vi "Fc_MenuSelections.vi"(6 "Cluster References":T2, 7 "ItemTag":string, 8 "error in (no error)":errorcluster, 9 "Cluster in":T1, 10 "VI caller":refnum<vi>, 11 "WaveformGraph in":refnum<vi>) -> (0 "error out":errorcluster, 3 "Cluster out":T1)   [LabVIEW 2021]
doc: "This function is used to select possible selection in the current window plot."
uses:
  <vilib>/Analysis/NI_AALBase.lvlib
  <vilib>/gmath/NI_Gmath.lvlib
  <vilib>/Analysis/1siggen.llb/Ramp Pattern by Samples.vi
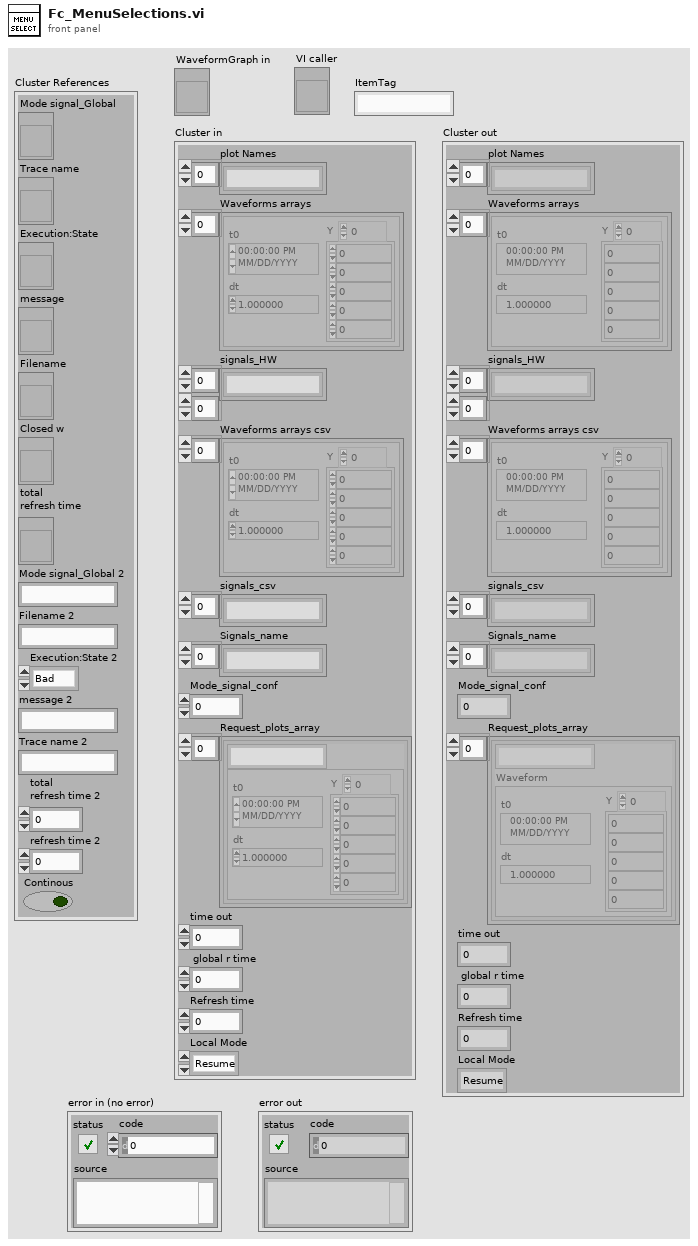
[diagram p1: front panel]
types:
  T1 = cluster{"plot Names":string[], "Waveforms arrays":waveform(dbl)[], "signals_HW":string[][], "Waveforms arrays csv":waveform(dbl)[], "signals_csv":string[], "Signals_name":string[], "Mode_signal_conf":u8, "Request_plots_array":cluster{string, "Waveform":waveform(dbl)}[], "time out":i32, " global r time":u32, "Refresh time":u32, "Local Mode":enum32{"Resume", "Hold"}}
  T2 = cluster{"Mode signal_Global":refnum<vi>, "Trace name":refnum<vi>, "Execution:State":refnum<vi>, "message":refnum<vi>, "Filename":refnum<vi>, "Closed w":refnum<vi>, "total \nrefresh time":refnum<vi>, "Mode signal_Global 2":string, "Filename 2":string, "Execution:State 2":enum32{"Bad", "Idle", "Run top level", "Running"}, "message 2":string, "Trace name 2":string, "total \nrefresh time 2":i32, "refresh time 2":i32, "Continous":bool}
  T3 = enum32{"Bad", "Idle", "Run top level", "Running"}
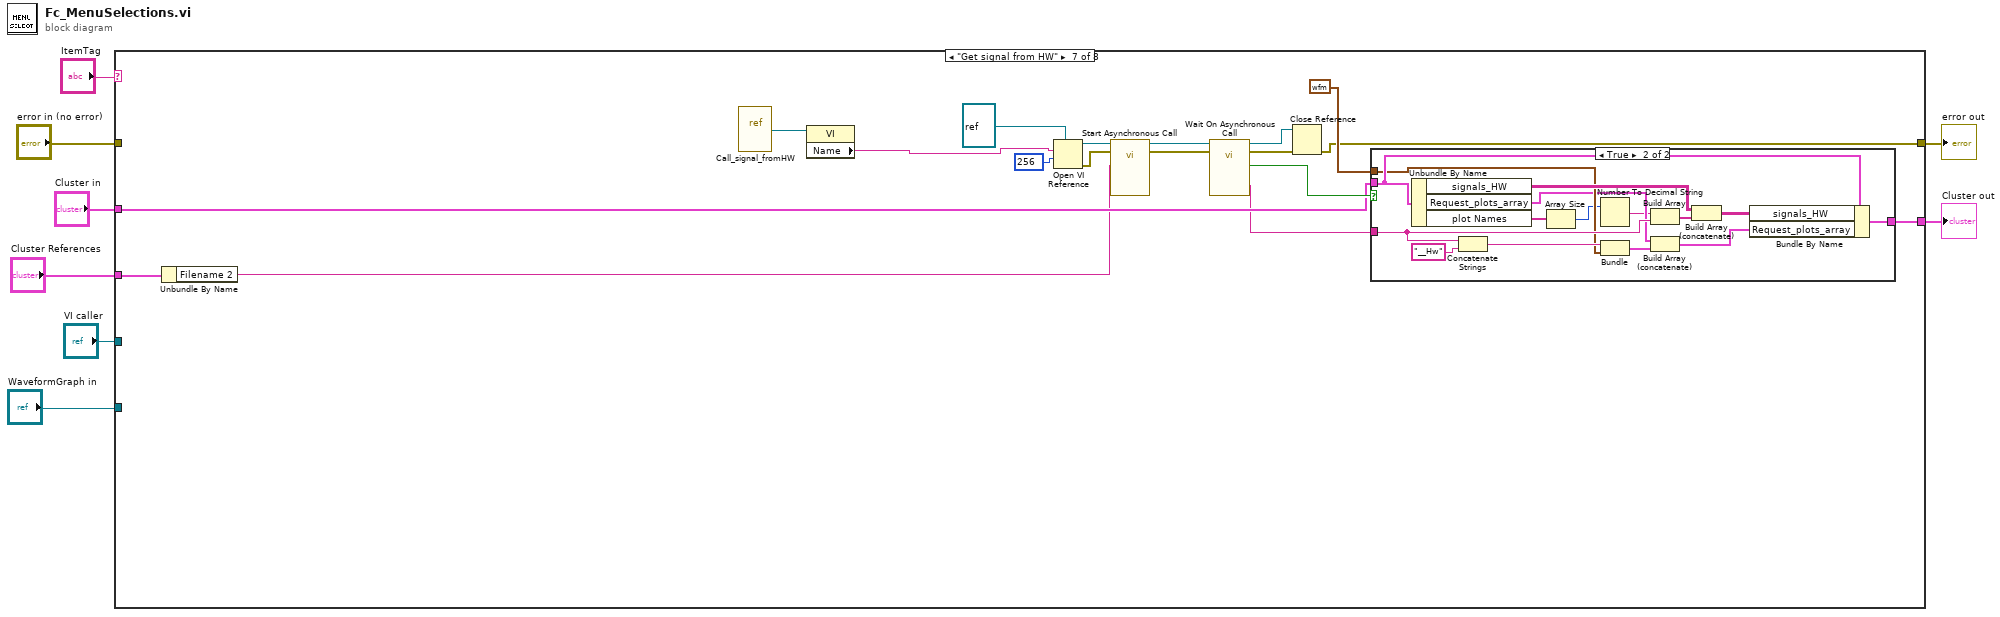
[diagram p0: block diagram]
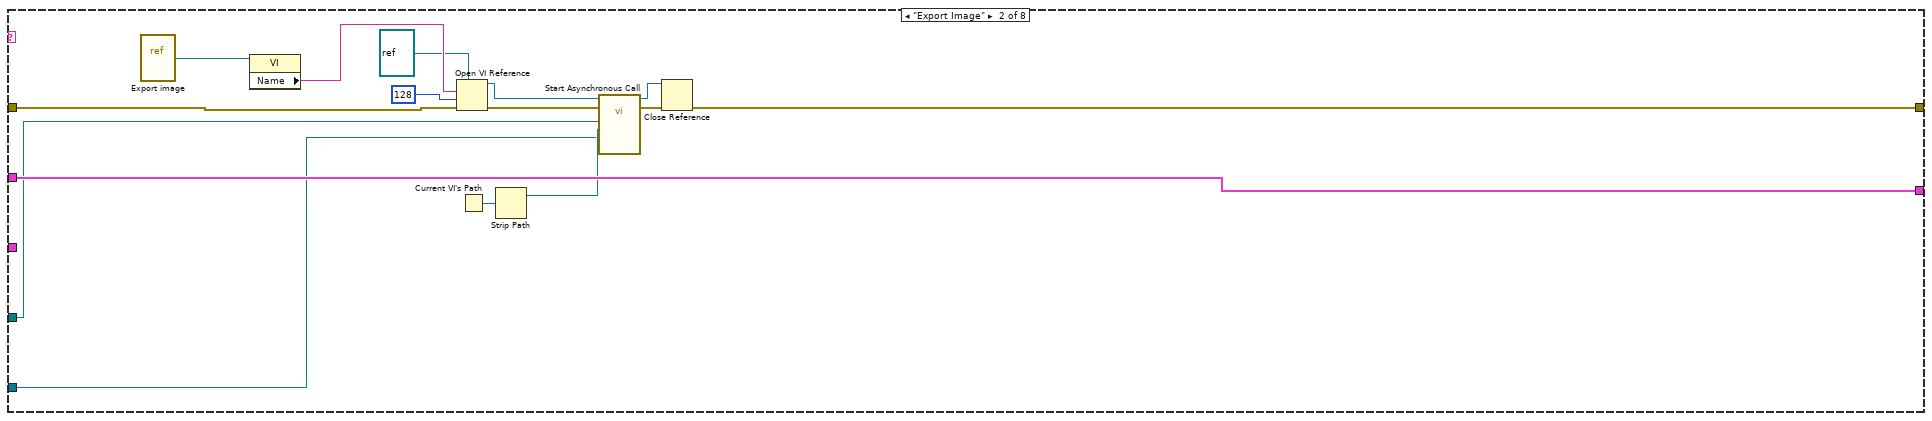
[diagram p3: hidden frame]
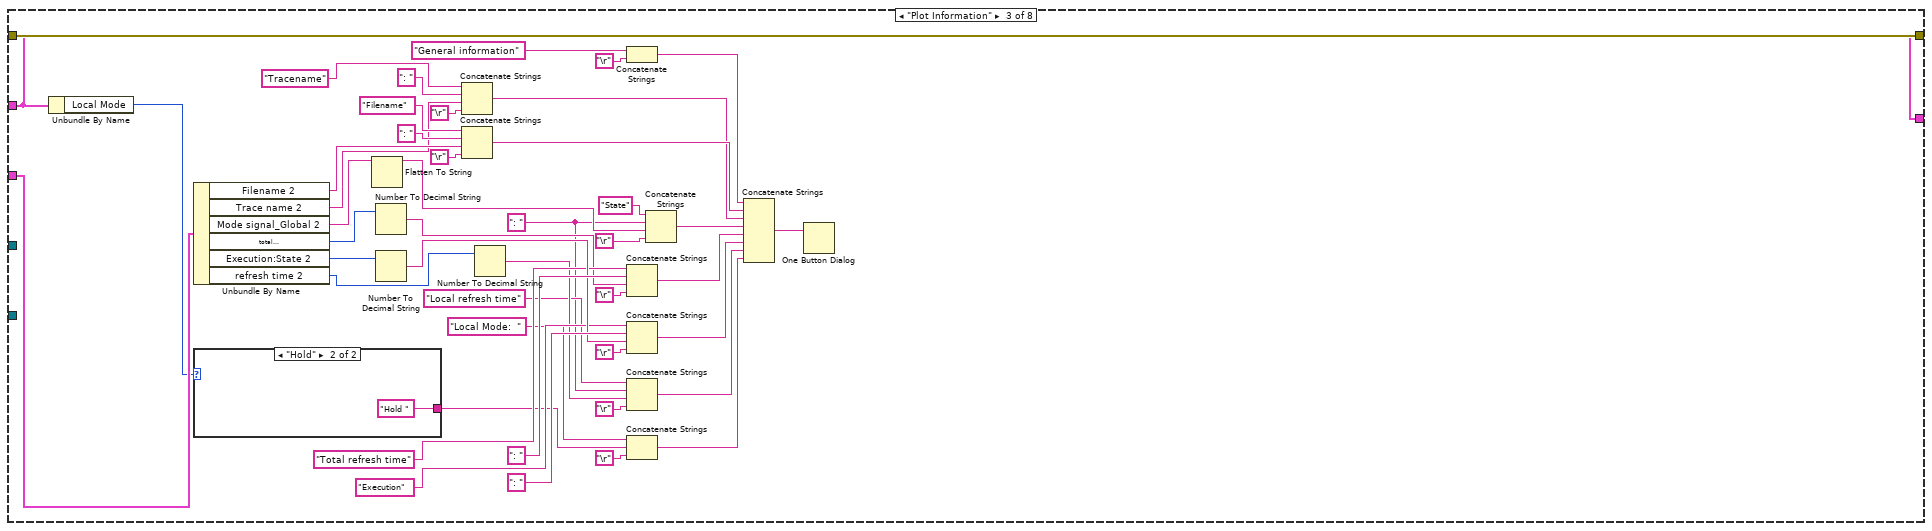
[diagram p4: hidden frame]
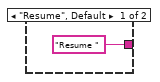
[diagram p5: hidden frame]
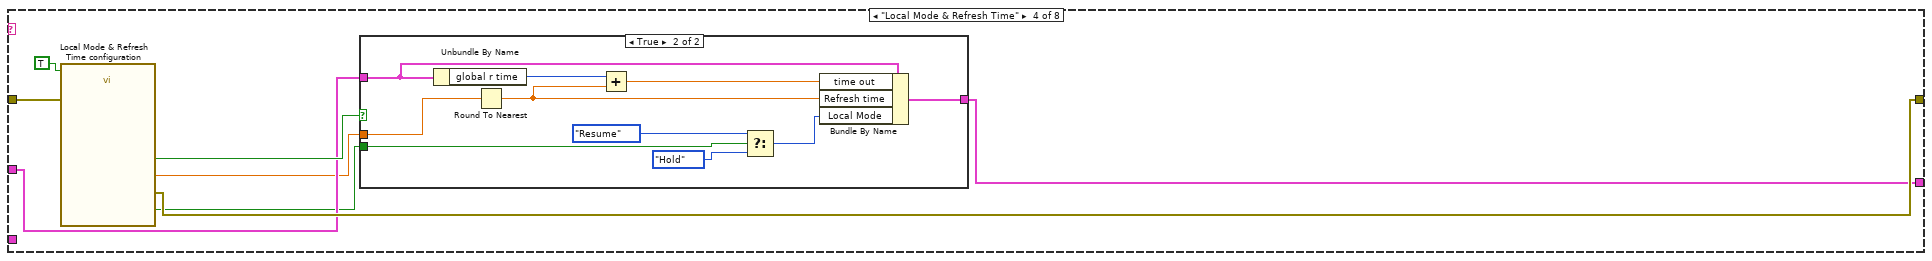
[diagram p6: hidden frame]
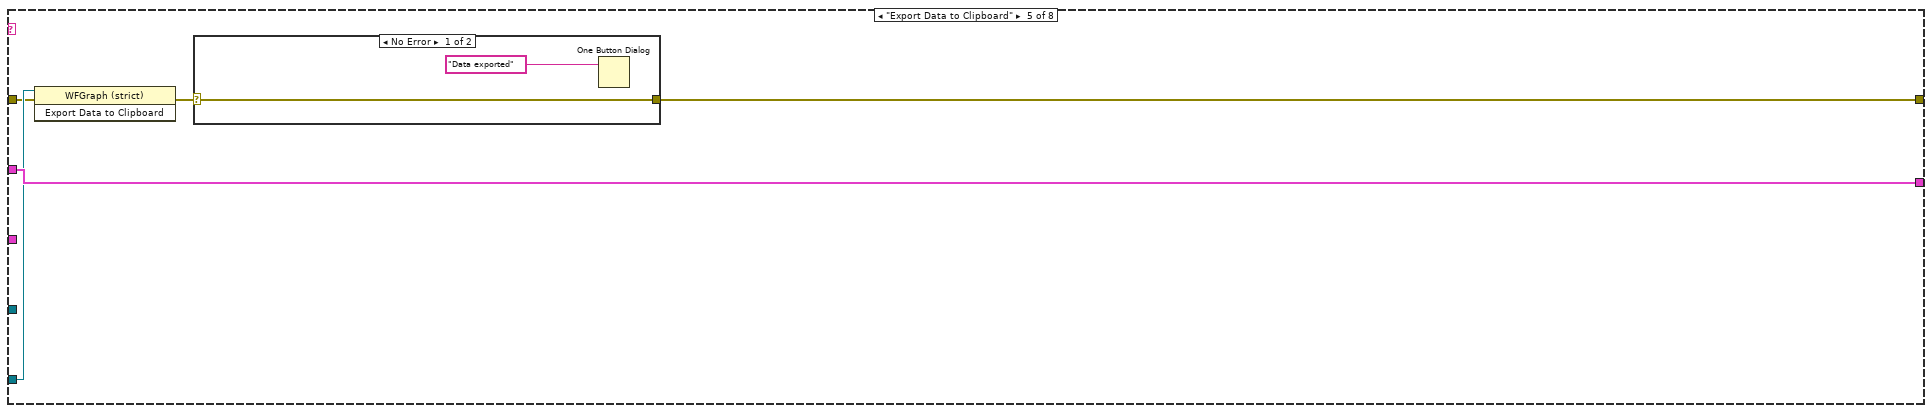
[diagram p8: hidden frame]
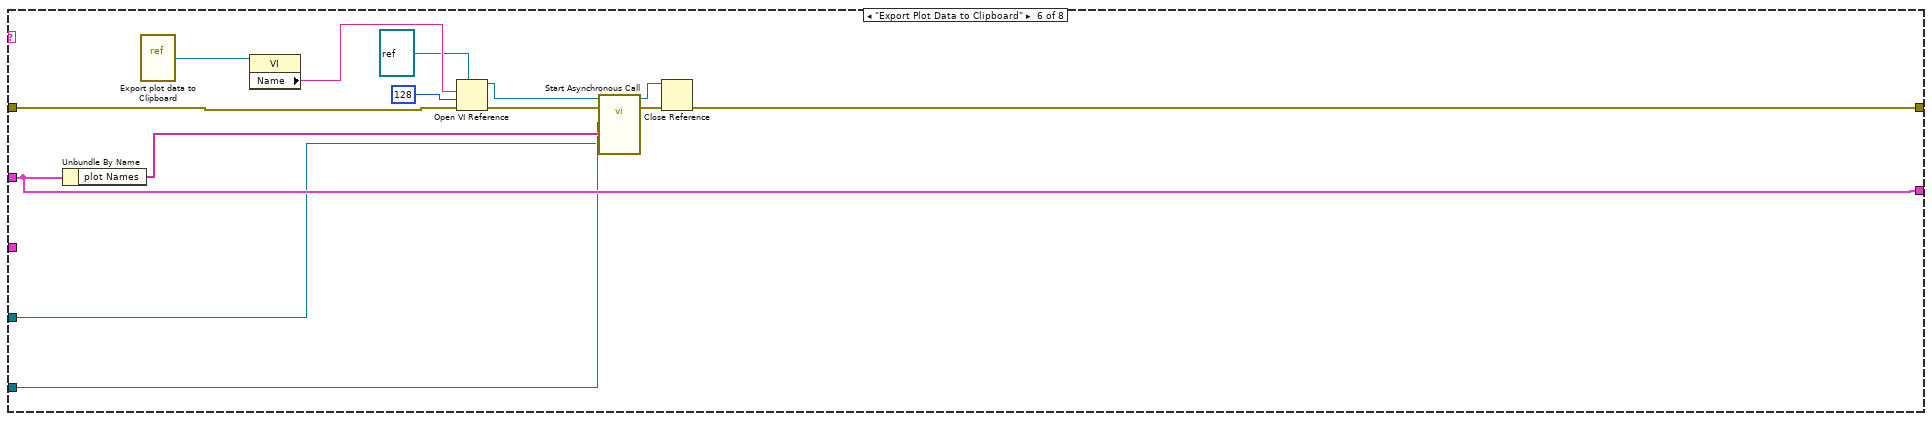
[diagram p10: hidden frame]
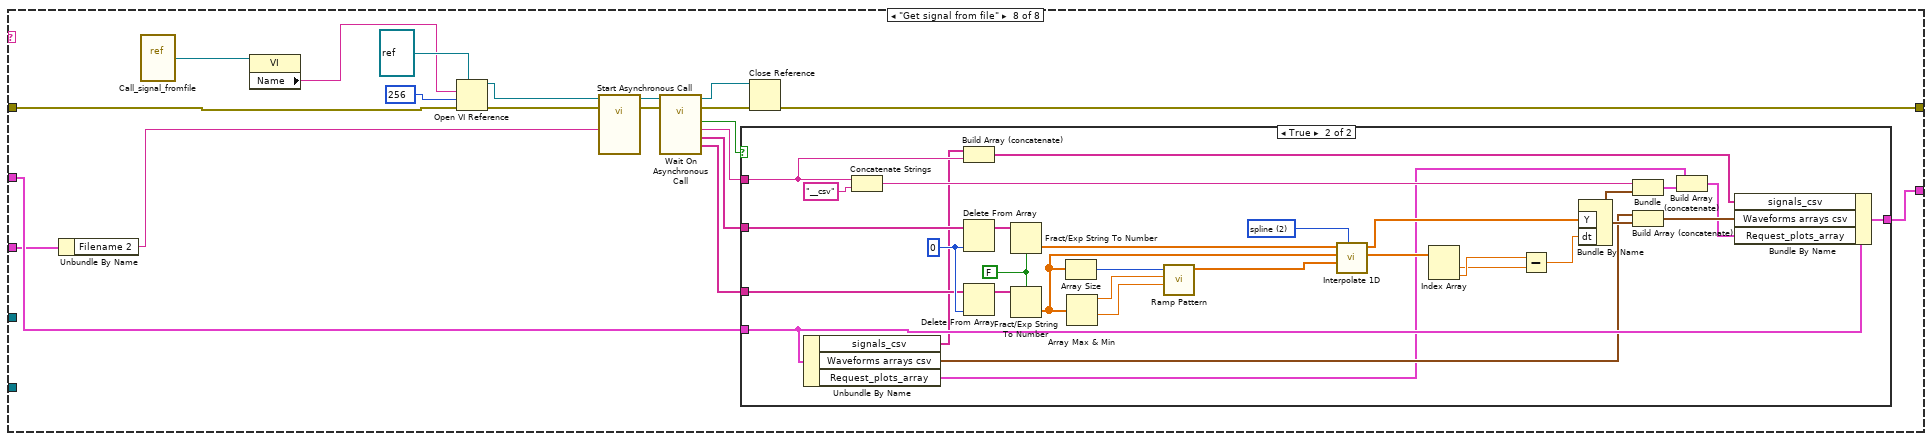
[diagram p12: hidden frame]
diagram:
  n1 = case shown="\"Get signal from HW\"" "ItemTag" {
    tunnel: [w10 w25 w31 w74 w96 w107 w127 w161] -> w4
    tunnel: "Cluster in" -> [w10 w25 w31 w76 w96 w107 w119 w162]
    tunnel: [w9 w14 w70 w78 w95 w103 w116 w151] -> w5
    tunnel: "error in (no error)" -> [w9 w13 w70 w79 w92 w102 _ w150]
    tunnel: "WaveformGraph in" -> [_ w12 _ _ w94 w101 _ _]
    tunnel: "VI caller" -> [_ w11 _ _ _ w100 _ _]
    tunnel: "Cluster References" -> [_ _ w69 _ _ _ w114 w149]
    frame "False", Default {
    }
    frame "Export Image" {
      n2 = vi-ref "Export image.vi"() -> (w19:refnum<vi>)
      n3 = property class="VI"(reference=w19) -> ("Name"=w21:string)  [unwired: 1 in, 2 out]
      n4 = Open VI Reference(type specifier VI Refnum (for type only)=refnum<vi> refnum ("reference"), vi path=w21, options=128, error in (no error)=w13) -> (vi reference=w22:refnum<vi>, error out=w23:errorcluster)  [unwired: 2 in]
      n5 = Current VI's Path() -> (path=w24:path)
      n6 = Strip Path(path=w24) -> (stripped path=w17:path)  [unwired: 1 out]
      n7 = call-by-ref "Start Asynchronous Call"(reference=w22, error in=w23, "Graph reference"=w12, "Folder selection"=w17, "VI caller"=w11) -> (reference out=w16:refnum<vi>, error out=w15:errorcluster)  [unwired: 8 in, 1 out]
      n8 = Close Reference(reference=w16, error in (no error)=w15) -> (error out=w14:errorcluster)
    }
    frame "Plot Information" {
      w33 = ": " ("string")
      n9 = Unbundle By Name(w31) -> ("Local Mode"=w30:enum32{"Resume", "Hold"})
      n10 = Unbundle By Name(w69) -> ("Filename 2"=w46:string, "Trace name 2"=w45:string, "Mode signal_Global 2"=w43:string, "total \nrefresh time 2"=w41:i32, "Execution:State 2"=w39:T3, "refresh time 2"=w35:i32)
      n11 = case shown="\"Hold\"" w30 {
        tunnel: ["Resume " ("string") "Hold " ("string")] -> w28
        frame "Resume", Default {
        }
        frame "Hold" {
        }
      }
      n12 = Flatten To String(anything=w43) -> (data string=w60:string)  [unwired: 3 in, 2 out]
      n13 = Number To Decimal String(number=w41) -> (decimal integer string=w40:string)  [unwired: 1 in]
      n14 = Number To Decimal String(number=w39) -> (decimal integer string=w53:string)  [unwired: 1 in]
      n15 = Concatenate Strings("Tracename" ("string"), ": " ("string"), w45, "\r") -> (w63:string)
      n16 = Concatenate Strings("Filename" ("string"), ": " ("string"), w46, "\r") -> (w64:string)
      n17 = Number To Decimal String(number=w35) -> (decimal integer string=w37:string)  [unwired: 1 in]
      n18 = Concatenate Strings("General information" ("string"), "\r") -> (w48:string)
      n19 = Concatenate Strings("Total refresh time" ("string"), ": " ("string"), w40, "\r") -> (w56:string)
      n20 = Concatenate Strings("Execution" ("string"), ": " ("string"), w53, "\r") -> (w52:string)
      n21 = Concatenate Strings("Local refresh time" ("Label.Text"), w33, w37, "\r") -> (w32:string)
      n22 = Concatenate Strings("Local Mode:  " ("string"), w28, "\r") -> (w26:string)
      n23 = Concatenate Strings("State" ("Label.Text"), w33, w60, "\r") -> (w59:string)
      n24 = Concatenate Strings(w48, w64, w63, w59, w56, w52, w32, w26) -> (w51:string)
      n25 = One Button Dialog(message=w51) -> ()  [unwired: 1 in, 1 out]
    }
    frame "Local Mode & Refresh Time" {
      n26 = call "Local Mode & Refresh Time configuration"("Enable"=TRUE, "error in (no error)"=w79) -> ("Refresh time"=w75:dbl, "Resume getting data"=w73:bool, "OK"=w77:bool, "error out"=w78:errorcluster)  [unwired: 14 in]
      n27 = case shown="True" w77 {
        tunnel: w76 -> [w81 w87]
        tunnel: w75 -> [_ w90]
        tunnel: [w81 w86] -> w74
        tunnel: w73 -> [_ w85]
        frame False {
        }
        frame True {
          n28 = Unbundle By Name(w87) -> ("global r time"=w91:u32)
          n29 = Round To Nearest(number=w90) -> (nearest integer value=w89:dbl)
          n30 = Add(x=w91, y=w89) -> (x+y=w88:dbl)
          n31 = Select(t=enum32{"Resume", "Hold"}."Resume" ("Local Mode"), s=w85, f=enum32{"Resume", "Hold"}."Hold" ("Local Mode")) -> (s? t:f=w82:enum32{"Resume", "Hold"})
          n32 = Bundle By Name(cluster=w87, "time out"=w88, "Refresh time"=w89, "Local Mode"=w82) -> (w86:T1)
        }
      }
    }
    frame "Export Data to Clipboard" {
      n33 = invoke class="WFGraph (strict)" method="Export Data to Clipboard"(reference=w94, error in=w92) -> (error out=w93:errorcluster)  [unwired: 1 in, 2 out]
      n34 = case shown="No Error" w93 {
        selector: w93 -> [w97 w99]
        tunnel: [w97 w99] -> w95
        frame No Error {
          n35 = One Button Dialog(message="Data exported") -> ()  [unwired: 1 in, 1 out]
        }
        frame Error {
        }
      }
    }
    frame "Export Plot Data to Clipboard" {
      n36 = Unbundle By Name(w107) -> ("plot Names"=w109:string[])
      n37 = vi-ref "Export plot data to Clipboard.vi"() -> (w104:refnum<vi>)
      n38 = property class="VI"(reference=w104) -> ("Name"=w113:string)  [unwired: 1 in, 2 out]
      n39 = Open VI Reference(type specifier VI Refnum (for type only)=refnum<vi> refnum ("reference"), vi path=w113, options=128, error in (no error)=w102) -> (vi reference=w112:refnum<vi>, error out=w111:errorcluster)  [unwired: 2 in]
      n40 = call-by-ref "Start Asynchronous Call"(reference=w112, error in=w111, "VI caller"=w100, "List Plots"=w109, "Graph reference"=w101) -> (reference out=w106:refnum<vi>, error out=w105:errorcluster)  [unwired: 2 in, 1 out]
      n41 = Close Reference(reference=w106, error in (no error)=w105) -> (error out=w103:errorcluster)
    }
    frame "Get signal from HW" {
      n42 = Unbundle By Name(w114) -> ("Filename 2"=w115:string)
      n43 = vi-ref "Call_signal_fromHW.vi"() -> (w128:refnum<vi>)
      n44 = property class="VI"(reference=w128) -> ("Name"=w120:string)  [unwired: 1 in, 2 out]
      n45 = Open VI Reference(type specifier VI Refnum (for type only)=refnum<vi> refnum ("reference"), vi path=w120, options=256) -> (vi reference=w129:refnum<vi>, error out=w131:errorcluster)  [unwired: 3 in]
      n46 = call-by-ref "Start Asynchronous Call"(reference=w129, error in=w131, "Plot window"=w115) -> (reference out=w125:refnum<vi>, error out=w126:errorcluster)  [unwired: 2 in, 3 out]
      n47 = call-by-ref "Wait On Asynchronous Call"(reference=w125, error in=w126) -> (reference out=w124:refnum<vi>, error out=w123:errorcluster, "Y name"=w117:string, "Ready?"=w122:bool)  [unwired: 3 in, 1 out]
      n48 = Close Reference(reference=w124, error in (no error)=w123) -> (error out=w116:errorcluster)
      n49 = case shown="True" w122 {
        tunnel: w117 -> [_ w146]
        tunnel: [w132 w141] -> w127
        tunnel: w119 -> [w132 w145]
        tunnel: waveform(dbl) {"t0"=timestamp(0 s since 1904-01-01), "dt"=1.0, "Y"=[]} ("Waveform") -> [_ w139]
        frame False {
        }
        frame True {
          n50 = Unbundle By Name(w145) -> ("signals_HW"=w144:string[][], "Request_plots_array"=w138:cluster{string, "Waveform":waveform(dbl)}[], "plot Names"=w135:string[])
          n51 = Concatenate Strings(w146, "__Hw" ("string")) -> (w140:string)
          n52 = Array Size(array=w135) -> (size(s)=w134:i32)
          n53 = Number To Decimal String(number=w134) -> (decimal integer string=w133:string)  [unwired: 1 in]
          n54 = Bundle(w140, "Waveform"=w139) -> (w137:cluster{string, "Waveform":waveform(dbl)})  [unwired: 1 in]
          n55 = Build Array(w133, w146) -> (w143:string[])
          n56 = Build Array (concatenate)(w138, w137) -> (w136:cluster{string, "Waveform":waveform(dbl)}[])
          n57 = Build Array (concatenate)(w144, w143) -> (w142:string[][])
          n58 = Bundle By Name(cluster=w145, "signals_HW"=w142, "Request_plots_array"=w136) -> (w141:T1)
        }
      }
    }
    frame "Get signal from file" {
      n59 = Unbundle By Name(w149) -> ("Filename 2"=w148:string)
      n60 = vi-ref "Call_signal_fromfile.vi"() -> (w165:refnum<vi>)
      n61 = property class="VI"(reference=w165) -> ("Name"=w159:string)  [unwired: 1 in, 2 out]
      n62 = Open VI Reference(type specifier VI Refnum (for type only)=refnum<vi> refnum, vi path=w159, options=256, error in (no error)=w150) -> (vi reference=w163:refnum<vi>, error out=w167:errorcluster)  [unwired: 2 in]
      n63 = call-by-ref "Start Asynchronous Call"(reference=w163, error in=w167, "Plot window"=w148) -> (reference out=w160:refnum<vi>, error out=w158:errorcluster)  [unwired: 3 in, 4 out]
      n64 = call-by-ref "Wait On Asynchronous Call"(reference=w160, error in=w158) -> (reference out=w153:refnum<vi>, error out=w152:errorcluster, "Y subarray"=w154:string[], "X subarray"=w155:string[], "Curve name"=w156:string, "Ready?"=w157:bool)  [unwired: 4 in]
      n65 = case shown="True" w157 {
        tunnel: w155 -> [_ w198]
        tunnel: w154 -> [_ w197]
        tunnel: w156 -> [_ w180]
        tunnel: w162 -> [w168 w174]
        tunnel: [w168 w175] -> w161
        frame False {
        }
        frame True {
          w189 = 2 items=["nearest", "linear", "spline", "cubic Hermite", "Lagrange"] ("method")
          w194 = FALSE ("use system decimal point (T)")
          w199 = 0 ("index")
          n66 = Unbundle By Name(w174) -> ("signals_csv"=w172:string[], "Waveforms arrays csv"=w173:waveform(dbl)[], "Request_plots_array"=w171:cluster{string, "Waveform":waveform(dbl)}[])
          n67 = Concatenate Strings(w180, "__csv" ("string")) -> (w179:string)
          n68 = Build Array (concatenate)(w172, w180) -> (w177:string[])
          n69 = Delete From Array(array=w198, index=w199) -> (array with subset deleted=w195:string[])  [unwired: 1 in, 1 out]
          n70 = Delete From Array(array=w197, index=w199) -> (array with subset deleted=w196:string[])  [unwired: 1 in, 1 out]
          n71 = Fract/Exp String To Number(use system decimal point (T)=w194, string=w195) -> (number=w186:dbl[])  [unwired: 2 in, 1 out]
          n72 = Fract/Exp String To Number(use system decimal point (T)=w194, string=w196) -> (number=w188:dbl[])  [unwired: 2 in, 1 out]
          n73 = Array Size(array=w188) -> (size(s)=w192:i32)
          n74 = Array Max & Min(array=w188) -> (max value=w191:dbl, min value=w190:dbl)  [unwired: 2 out]
          n75 = call-poly <vilib>:"Ramp Pattern.vi"("start"=w190, "end"=w191, "samples"=w192) -> ("Ramp Pattern"=w187:dbl[])  [unwired: 7 in, 1 out]
          n76 = call <vilib>:"Interpolate 1D.vi"("method"=w189, "xi"=w187, "X"=w188, "Y"=w186) -> ("xi used"=w185:dbl[], "yi"=w184:dbl[])  [unwired: 5 in, 1 out]
          n77 = Index Array(array=w185) -> (element #1=w182:dbl, element #2=w183:dbl)  [unwired: 2 in]
          n78 = Subtract(x=w183, y=w182) -> (x-y=w181:dbl)
          n79 = Bundle By Name("Y"=w184, "dt"=w181) -> (w178:waveform(dbl))  [unwired: 1 in]
          n80 = Bundle(w179, w178) -> (w170:cluster{string, waveform(dbl)})  [unwired: 1 in]
          n81 = Build Array (concatenate)(w173, w178) -> (w176:waveform(dbl)[])
          n82 = Build Array (concatenate)(w171, w170) -> (w169:cluster{string, "Waveform":waveform(dbl)}[])
          n83 = Bundle By Name(cluster=w174, "signals_csv"=w177, "Waveforms arrays csv"=w176, "Request_plots_array"=w169) -> (w175:T1)
        }
      }
      n84 = Close Reference(reference=w153, error in (no error)=w152) -> (error out=w151:errorcluster)
    }
  }
  "error out" <- w5
  "Cluster out" <- w4
